vi "Read Multiple Sections.vi"(7 "error in (no error)":errorcluster, 8 "Cluster of Section Clusters":variant, 10 "JSON Sections":string="{}") -> (0 "error out":errorcluster, 1 "Cluster out":variant)   [LabVIEW 2021, in "json.facade.lvlib"]
doc: "Set Multiple Sections from Sections of a JSON object. If the Section is not specified, then the data name of the Cluster will be used.\n\nA \"Section Cluster\" is defined in analogy to the OpenG Variant Config Library \"Section Cluster\" functions, using a JSON Object, with subObjects representing \"Sections\", instead of INI format."
uses:
  json.facade.lvlib
  jsontext/JSONtext.lvlib
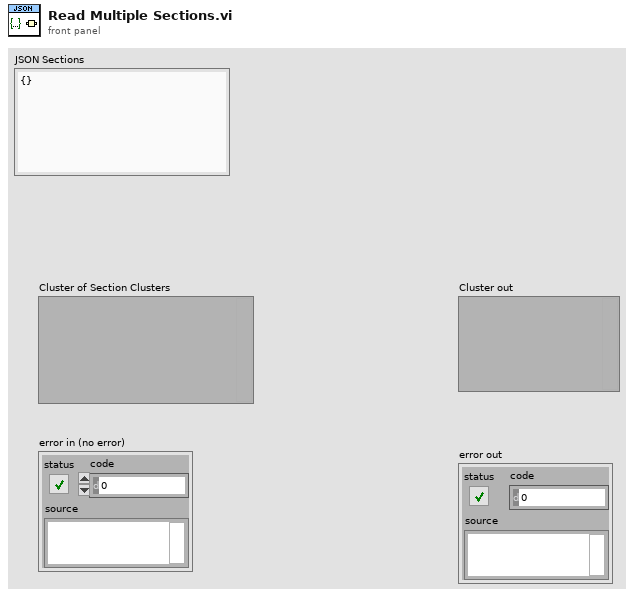
[diagram p1: front panel]
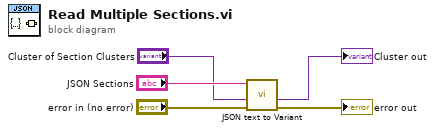
[diagram p0: block diagram]
diagram:
  n1 = call "JSON text to Variant.vi"("error in (no error)"="error in (no error)", "Data Type"="Cluster of Section Clusters", "JSON"="JSON Sections") -> ("error out"=→"error out":errorcluster, "Variant out"=→"Cluster out":variant)  [unwired: 7 in]
